vi "DSF.Engine.Transfer Group.Create.vi"(5 "Debug Flags":refnum<class "DSF.Engine.Debug Flags.lvclass">, 6 "transceiver id":i32, 7 "framework id":i32, 8 "error in (no error)":errorcluster, 9 "Direction":T1, 10 "Timing":refnum<class "DSF.Engine.Timing.lvclass">, 11 "Transfers":refnum<class "DSF.Engine.Transfer.lvclass">[](array[class])) -> (0 "error out":errorcluster, 3 "Transfer Group out":refnum<class "DSF.Engine.Transfer Group.lvclass">)   [LabVIEW 2017, in "DSF.Engine.lvlib" / "DSF.Engine.Transfer Group.lvclass"]
uses:
  DSF.Engine.Transfer Group.lvclass
  DSF.Engine.Transfer.lvclass
  Timing/DSF.Engine.Timing.lvclass
  DSF Configuration API/1.0.0/Public/Controls/DSF Direction.ctl
  Debug/DSF.Engine.Debug Flags.lvclass
  DSF.Engine.Transfer Group.lvclass/DSF.Engine.Transfer Group.ctl
  DSF Configuration API/1.0.0/DSF Configuration API.lvlib
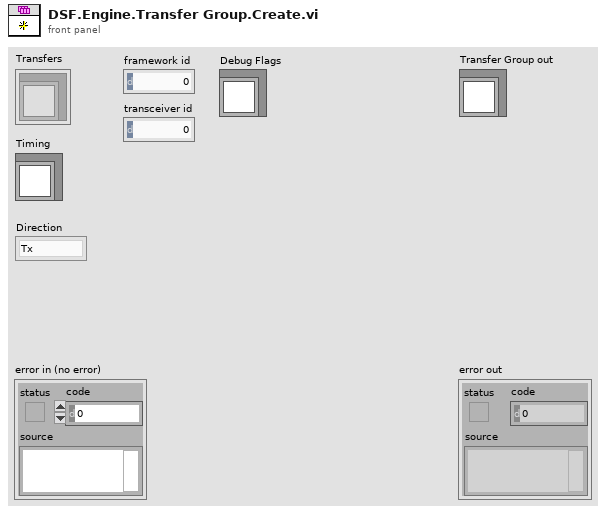
[diagram p1: front panel]
types:
  T1 = typedef "DSF Configuration API.lvlib/DSF Direction.ctl" = enum8{"Tx", "Rx"}
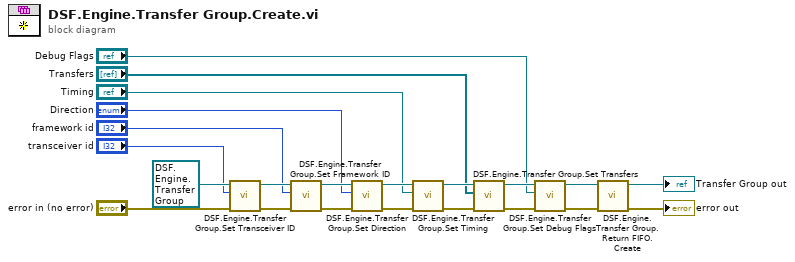
[diagram p0: block diagram]
diagram:
  n1 = call "DSF.Engine.Transfer Group.Set Transceiver ID.vi"("transceiver id"="transceiver id", "Transfer Group in"=refnum<class "DSF.Engine.Transfer Group.lvclass"> refnum ("Transfer Group type")) -> ("Transfer Group out"=w4:refnum<class "DSF.Engine.Transfer Group.lvclass">)  [unwired: 9 in]
  n2 = call "DSF.Engine.Transfer Group.Set Framework ID.vi"("framework id"="framework id", "Transfer Group in"=w4) -> ("Transfer Group out"=w16:refnum<class "DSF.Engine.Transfer Group.lvclass">)  [unwired: 9 in]
  n3 = call "DSF.Engine.Transfer Group.Set Direction.vi"("Direction"="Direction", "Transfer Group in"=w16) -> ("Transfer Group out"=w15:refnum<class "DSF.Engine.Transfer Group.lvclass">)  [unwired: 9 in]
  n4 = call "DSF.Engine.Transfer Group.Set Timing.vi"("Timing"="Timing", "Transfer Group in"=w15) -> ("Transfer Group out"=w14:refnum<class "DSF.Engine.Transfer Group.lvclass">)  [unwired: 9 in]
  n5 = call "DSF.Engine.Transfer Group.Set Transfers.vi"("Transfers"="Transfers", "Transfer Group in"=w14) -> ("Transfer Group out"=w7:refnum<class "DSF.Engine.Transfer Group.lvclass">)  [unwired: 9 in]
  n6 = call "DSF.Engine.Transfer Group.Set Debug Flags.vi"("Debug Flags"="Debug Flags", "Transfer Group in"=w7) -> ("Transfer Group out"=w6:refnum<class "DSF.Engine.Transfer Group.lvclass">)  [unwired: 9 in]
  n7 = call "DSF.Engine.Transfer Group.Return FIFO.Create.vi"("error in (no error)"="error in (no error)", "Transfer Group in"=w6) -> ("error out"=→"error out":errorcluster, "Transfer Group out"=→"Transfer Group out":refnum<class "DSF.Engine.Transfer Group.lvclass">)  [unwired: 8 in]
